vi "GlobalClicksHeight_flt.vi"() -> ()   [LabVIEW 2019]
panel:
  in  "Starting Height (nm)":dbl
  out "Setpoint (A)":dbl=100.0
  out "Current (pA)":dbl
  in  "Found Surface?":bool
  out "Surface Location":dbl
  in  "Starting Height?":bool
  in  "Clicks and Height":bool
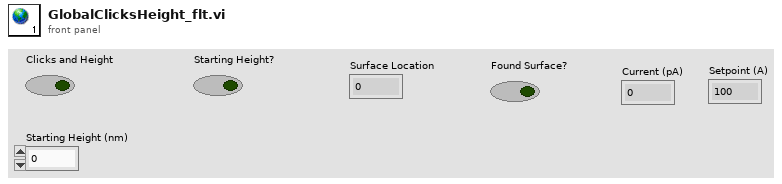
[diagram p1: front panel]
diagram:
